vi "Test HighFrequency Client Connection.vi"() -> ()   [LabVIEW 2013]
uses:
  <vilib>/LabVIEW Open Source Project/MQTT Control Packets/Control Packets/CONNACK/Connect Return Code -- enum.ctl
  source/Server class/Server.lvclass/Server.ctl
  <vilib>/LabVIEW Open Source Project/MQTT Client/Client class/Client.lvclass/Client.ctl
  <vilib>/LabVIEW Open Source Project/MQTT Control Packets/Control Packets/PUBLISH/PUBLISH.lvclass
  source/Server class/Server.lvclass
  <vilib>/LabVIEW Open Source Project/MQTT Connection/MQTT_Base/Base Class/MQTT_Base.lvclass
  <vilib>/LabVIEW Open Source Project/MQTT Client/Client class/Client.lvclass
  <vilib>/LabVIEW Open Source Project/MQTT TCP Connection/MQTT_TCP/Connection/TCPConnection.lvclass
  <vilib>/LabVIEW Open Source Project/MQTT Control Packets/Control Packets/CONNACK/CONNACK.lvclass
panel:
  out "Start timed out":bool
  out "NO RESPONSE":bool
  out "Stop timed out?":bool
  out "Stop":dbl format="%.06f"
  out "Connect":dbl format="%.06f"
  out "Start":dbl format="%.06f"
  out "STOPPING":bool
  out "Waveform Chart":T1(graph)
  out "Loop period (s)":dbl format="%.06f"
  out "client Outgoing ID Request":i32
  out "Process Response":i32
  out "Process Incoming ID Request":i32
  out "Process Status":T2=enum."Server Unavailable"
  out "error server":errorcluster
  out "Client Status":T2=enum."Server Unavailable"
  out "error client process":errorcluster
  out "NbConnections":u32
  out "error client consumer":errorcluster
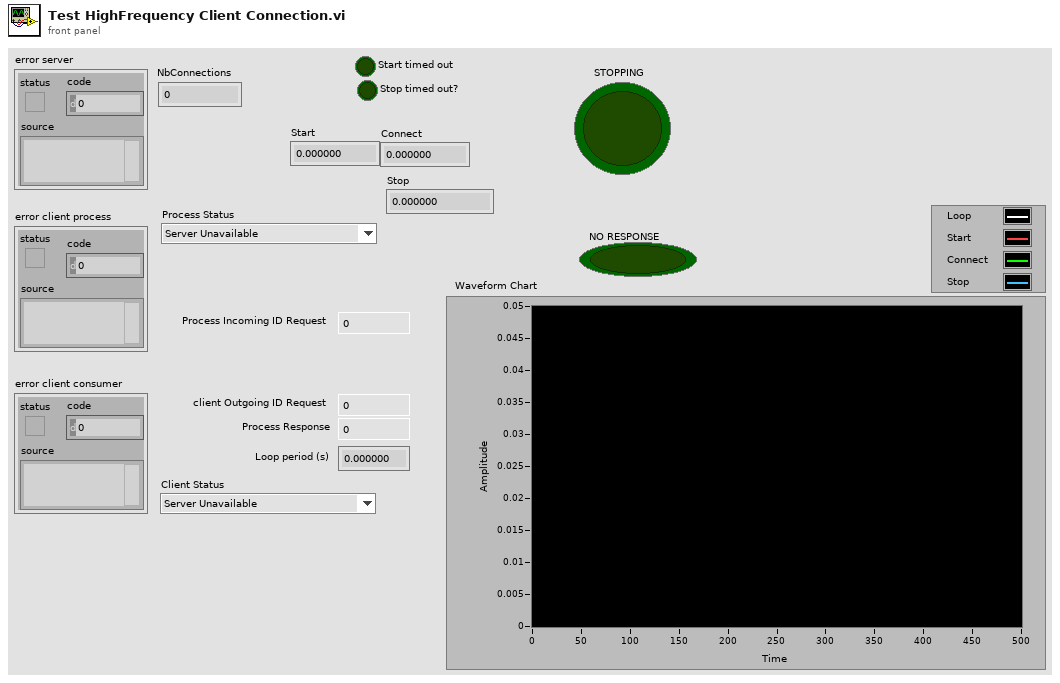
[diagram p1: front panel]
types:
  T1 = cluster{dbl, "elapsed (s)":dbl, "elapsed (s)":dbl, "elapsed (s)":dbl}
  T2 = typedef "MQTT_Control_Packets.lvlib/CONNACK.lvclass/Connect Return Code -- enum.ctl" = enum16{"Connection accepted", "Unacceptable protocol version", "Identifier Rejected", "Server Unavailable", "Bad Username or Password", "Not Authorized"}
  T3 = cluster{dbl, "elapsed (s)":dbl, "elapsed (s)":dbl, "elapsed (s)":dbl}[]
  T4 = typedef "MQTT Server.lvlib/Server.lvclass/Public Events -- cluster.ctl" = cluster{"NbConnections":refnum<user-event>}
  T5 = typedef "MQTT Client.lvlib/Client.lvclass/Public Events -- cluster.ctl" = cluster{"Connection Status":refnum<user-event>, "Connected":refnum<user-event>, "Application Message":refnum<user-event>}
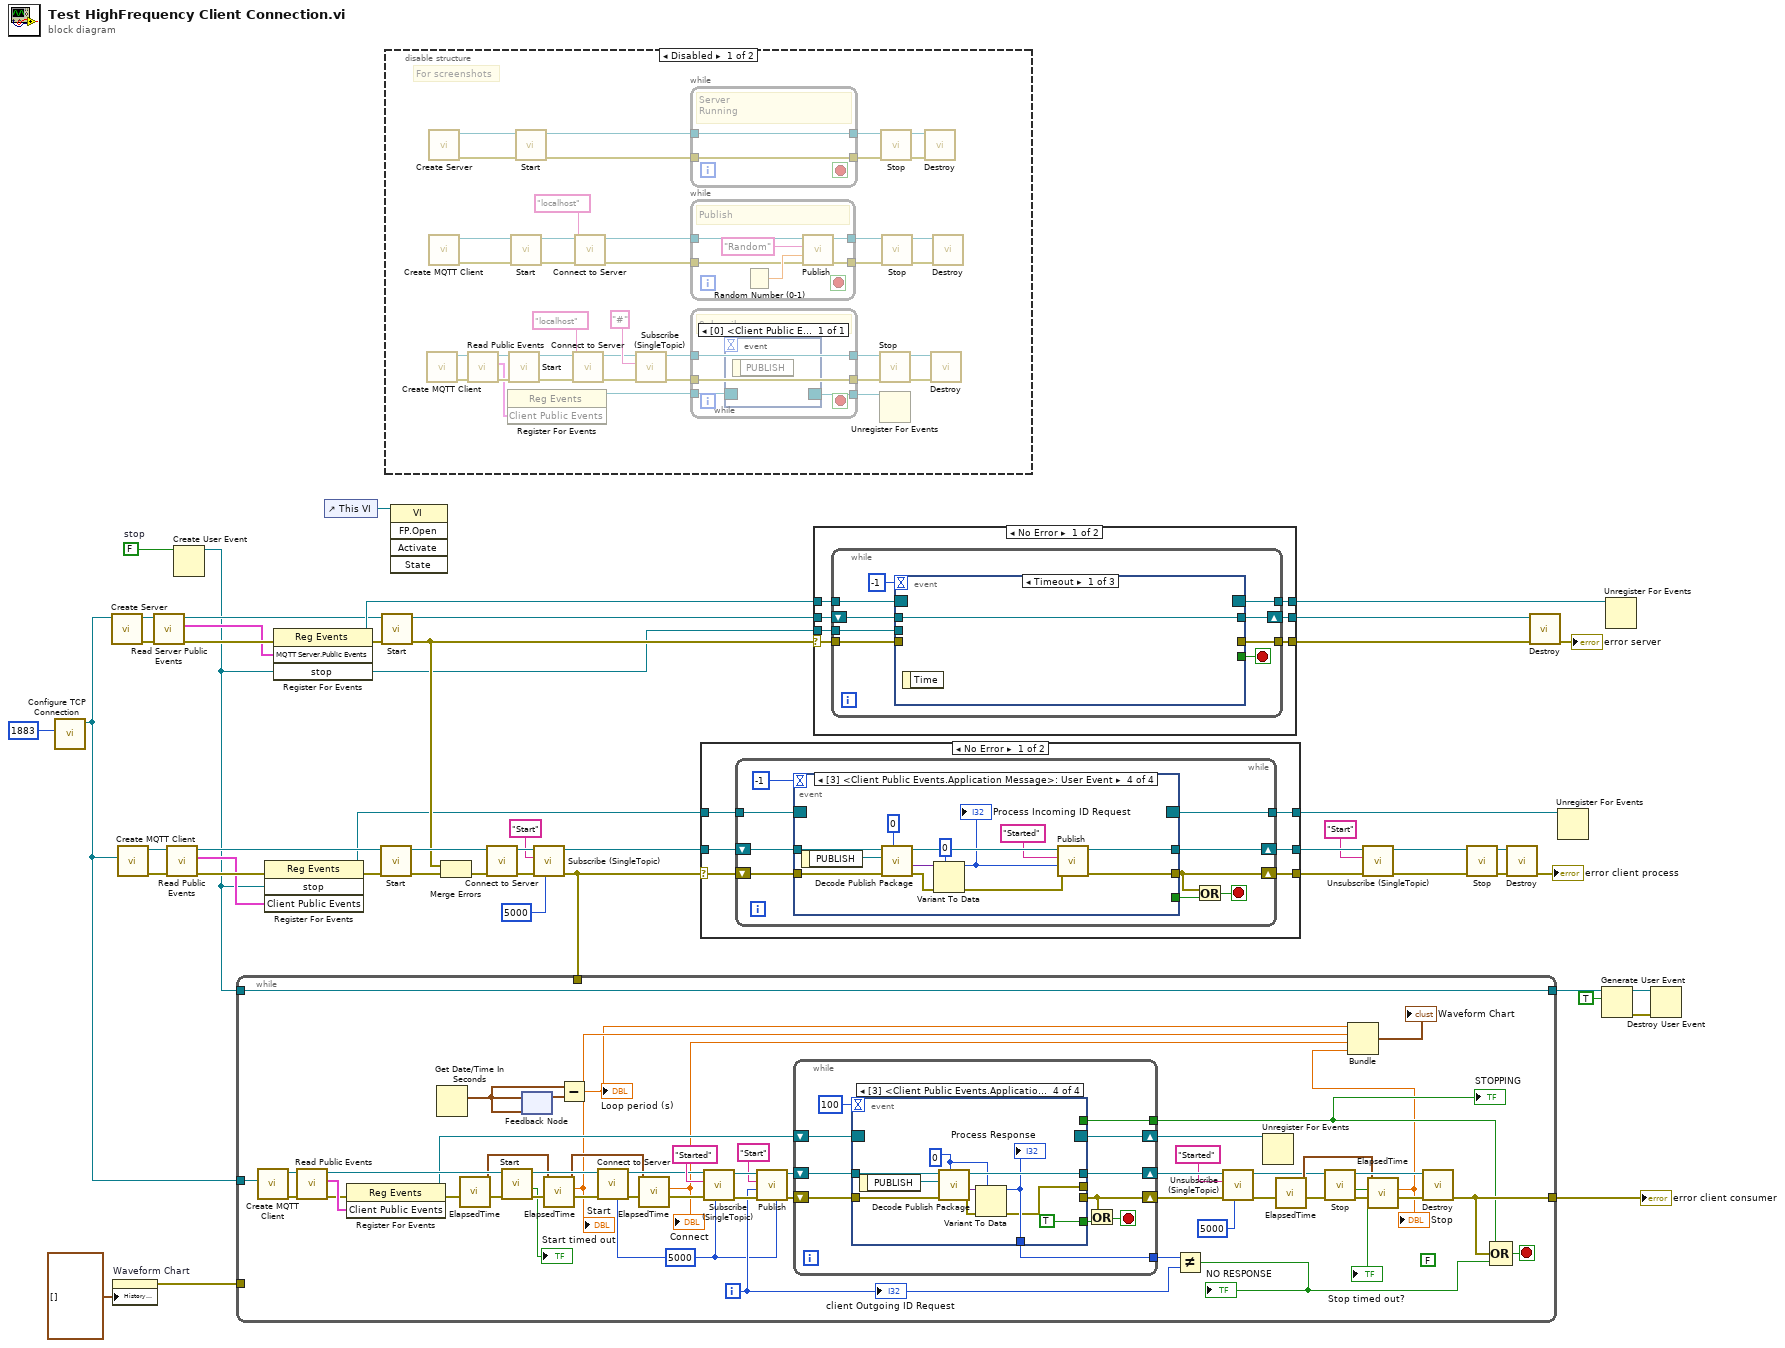
[diagram p0: block diagram]
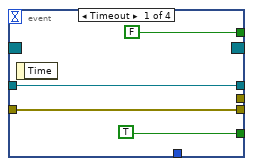
[diagram p2: hidden frame]
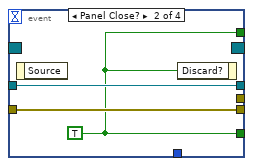
[diagram p3: hidden frame]
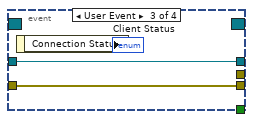
[diagram p4: hidden frame]
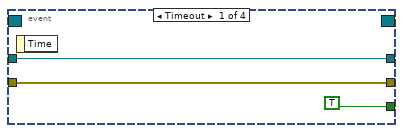
[diagram p5: hidden frame]
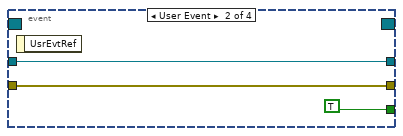
[diagram p6: hidden frame]
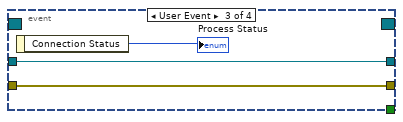
[diagram p7: hidden frame]
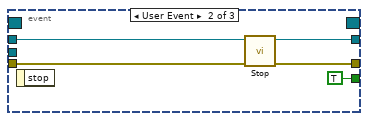
[diagram p10: hidden frame]
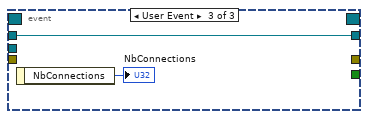
[diagram p11: hidden frame]
diagram:
  w33 = FALSE  # stop
  n1 = call <vilib>:"Configure TCP Connection.vi"("remote port (80)"=u16 1883) -> ("TCPConnection"=w2:refnum<class "TCPConnection.lvclass">)  [unwired: 9 in, 1 out]
  n2 = call "Create Server.vi"("Connection Configuration"=w2) -> ("error out"=w48:errorcluster, "Server"=w49:refnum<class "Server.lvclass">)  [unwired: 9 in]
  n3 = property on="Waveform Chart" class="WFChart (strict)"("History Data"=T3 []) -> (error out=w4:errorcluster)  [unwired: 2 in, 1 out]
  n4 = call <vilib>:"Create MQTT Client.vi"("Connection Configuration"=w2) -> ("error out"=w38:errorcluster, "Client out"=w37:refnum<class "Client.lvclass">)  [unwired: 9 in]
  n5 = call "Read Server Public Events.vi"("error in (no error)"=w48, "Server in"=w49) -> ("error out"=w47:errorcluster, "MQTT Server.Public Events"=w46:T4, "Server out"=w43:refnum<class "Server.lvclass">)  [unwired: 7 in]
  n6 = call <vilib>:"Read Public Events.vi"("error in (no error)"=w38, "Client in"=w37) -> ("error out"=w32:errorcluster, "Client Public Events"=w30:T5, "Client out"=w36:refnum<class "Client.lvclass">)  [unwired: 7 in]
  n7 = Create User Event(user event datatype=w33) -> (user event=w10:refnum<user-event>)  [unwired: 1 in, 1 out]
  n8 = register-events(error in=w32, w10, w30) -> (reference out=w22:refnum<event-registration>, error out=w31:errorcluster)  [unwired: 1 in]
  n9 = register-events(error in=w47, w46, w10) -> (reference out=w45:refnum<event-registration>, error out=w41:errorcluster)  [unwired: 1 in]
  n10 = control-ref of="This VI"() -> (w29:refnum<vi>)
  n11 = call <vilib>:"Start.vi"("error in (no error)"=w31, "MQTT_Base in"=w36) -> ("error out"=w34:errorcluster, "MQTT_Base out"=w35:refnum<class "Client.lvclass">)  [unwired: 7 in, 1 out]
  n12 = call <vilib>:"Start.vi"("error in (no error)"=w41, "MQTT_Base in"=w43) -> ("error out"=w27:errorcluster, "MQTT_Base out"=w42:refnum<class "Server.lvclass">)  [unwired: 7 in, 1 out]
  n13 = disable-structure shown="Disabled" {
    frame Disabled {
      # "For screenshots"
      n14 = call <vilib>:"Create MQTT Client.vi"() -> ("error out"=w55:errorcluster, "Client out"=w57:refnum<class "Client.lvclass">)  [unwired: 10 in]
      n15 = call "Create Server.vi"() -> ("error out"=w82:errorcluster, "Server"=w81:refnum<class "Server.lvclass">)  [unwired: 10 in]
      n16 = call <vilib>:"Create MQTT Client.vi"() -> ("error out"=w79:errorcluster, "Client out"=w80:refnum<class "Client.lvclass">)  [unwired: 10 in]
      n17 = call <vilib>:"Read Public Events.vi"("error in (no error)"=w55, "Client in"=w57) -> ("error out"=w54:errorcluster, "Client Public Events"=w53:T5, "Client out"=w56:refnum<class "Client.lvclass">)  [unwired: 7 in]
      n18 = register-events(w53) -> (reference out=w52:refnum<event-registration>)  [unwired: 2 in, 1 out]
      n19 = call <vilib>:"Start.vi"("error in (no error)"=w54, "MQTT_Base in"=w56) -> ("error out"=w72:errorcluster, "MQTT_Base out"=w73:refnum<class "Client.lvclass">)  [unwired: 7 in, 1 out]
      n20 = call <vilib>:"Start.vi"("error in (no error)"=w79, "MQTT_Base in"=w80) -> ("error out"=w86:errorcluster, "MQTT_Base out"=w85:refnum<class "Client.lvclass">)  [unwired: 7 in, 1 out]
      n21 = call <vilib>:"Start.vi"("error in (no error)"=w82, "MQTT_Base in"=w81) -> ("error out"=w64:errorcluster, "MQTT_Base out"=w66:refnum<class "Server.lvclass">)  [unwired: 7 in, 1 out]
      n22 = call <vilib>:"Connect to Server.vi"("error in (no error)"=w72, 10:"localhost" ("Topic Filter"), "Client in"=w73) -> ("error out"=w60:errorcluster, "Client out"=w61:refnum<class "Client.lvclass">)  [unwired: 5 in, 2 out]
      n23 = call <vilib>:"Connect to Server.vi"("error in (no error)"=w86, 10:"localhost" ("Topic Filter"), "Client in"=w85) -> ("error out"=w68:errorcluster, "Client out"=w71:refnum<class "Client.lvclass">)  [unwired: 5 in, 2 out]
      n24 = call <vilib>:"Subscribe (SingleTopic).vi"("error in (no error)"=w60, "Topic Filter"="#", "MQTT_Base in"=w61) -> ("error out"=w58:errorcluster, "MQTT_Base out"=w59:refnum<class "Client.lvclass">)  [unwired: 6 in, 1 out]
      n25 = while {
        tunnel: [w100] -> w67
        tunnel: w66 -> [w100]
        tunnel: w64 -> [w99]
        tunnel: [w99] -> w65
        stop <- _ stop-if-true
        # "Server\nRunning"
      }
      n26 = while {
        tunnel: w71 -> [w96]
        tunnel: [w95] -> w70
        tunnel: [w94] -> w69
        tunnel: w68 -> [w93]
        stop <- _ stop-if-true
        # "Publish"
        n27 = Random Number (0-1)() -> (number: 0 to 1=w98:dbl)
        n28 = call <vilib>:"Publish.vi"("error in (no error)"=w93, "Payload"=w98, "Topic Name (empty: Payload name)"="Random", "Client in"=w96) -> ("error out"=w94:errorcluster, "Client out"=w95:refnum<class "Client.lvclass">)  [unwired: 5 in, 1 out]
      }
      n29 = while {
        tunnel: [w92] -> w62
        tunnel: w59 -> [w92]
        tunnel: w58 -> [w91]
        tunnel: [w91] -> w63
        tunnel: w52 -> [w90]
        tunnel: [w89] -> w51
        stop <- _ stop-if-true
        # "Subscribe"
        n30 = event shown="[0] <Client Public Events.Application Message>: User Event" {
          selector: w90 -> [_]
          dyn-events: [_] -> w89
          timeout: _ -> [_]
          event User Event {
            n31 = event-data() -> ()  [unwired: 1 in, 1 out]
          }
        }
      }
      n32 = call <vilib>:"Stop.vi"("error in (no error)"=w63, "MQTT_Base in"=w62) -> ("error out"=w75:errorcluster, "MQTT_Base out"=w76:refnum<class "Client.lvclass">)  [unwired: 7 in, 1 out]
      n33 = Unregister For Events(event registration refnum=w51) -> ()  [unwired: 1 in, 1 out]
      n34 = call <vilib>:"Stop.vi"("error in (no error)"=w65, "MQTT_Base in"=w67) -> ("error out"=w88:errorcluster, "MQTT_Base out"=w87:refnum<class "Server.lvclass">)  [unwired: 7 in, 1 out]
      n35 = call <vilib>:"Stop.vi"("error in (no error)"=w69, "MQTT_Base in"=w70) -> ("error out"=w84:errorcluster, "MQTT_Base out"=w83:refnum<class "Client.lvclass">)  [unwired: 7 in, 1 out]
      n36 = call <vilib>:"Destroy.vi"("error in (no error)"=w88, "MQTT_Base in"=w87) -> ()  [unwired: 8 in, 2 out]
      n37 = call <vilib>:"Destroy.vi"("error in (no error)"=w75, "MQTT_Base in"=w76) -> ()  [unwired: 8 in, 2 out]
      n38 = call <vilib>:"Destroy.vi"("error in (no error)"=w84, "MQTT_Base in"=w83) -> ()  [unwired: 8 in, 2 out]
    }
    frame Enabled {
    }
  }
  n39 = invoke class="VI" method="FP.Open"(reference=w29) -> ()  [unwired: 4 in, 5 out]
  n40 = Merge Errors(w27, w34) -> (w39:errorcluster)
  n41 = call <vilib>:"Connect to Server.vi"("error in (no error)"=w39, "Client in"=w35) -> ("error out"=w25:errorcluster, "Client out"=w26:refnum<class "Client.lvclass">)  [unwired: 6 in, 2 out]
  n42 = call <vilib>:"Subscribe (SingleTopic).vi"("timeout (100ms)"=5000, "error in (no error)"=w25, "Topic Filter"="Start", "MQTT_Base in"=w26) -> ("error out"=w11:errorcluster, "MQTT_Base out"=w23:refnum<class "Client.lvclass">)  [unwired: 5 in, 1 out]
  n43 = while {
    tunnel: [w134] -> w12
    tunnel: w11 -> [_]
    tunnel: [w132] -> w9
    tunnel: w10 -> [w132]
    tunnel: w4 -> [_]
    tunnel: w2 -> [w104]
    i -> [w133]
    stop <- w135 stop-if-true
    w103 = 5000 ("timeout (100ms)")
    (unwired) FALSE
    n44 = call <vilib>:"Create MQTT Client.vi"("Connection Configuration"=w104) -> ("error out"=w151:errorcluster, "Client out"=w152:refnum<class "Client.lvclass">)  [unwired: 9 in]
    n45 = call <vilib>:"Read Public Events.vi"("error in (no error)"=w151, "Client in"=w152) -> ("error out"=w146:errorcluster, "Client Public Events"=w147:T5, "Client out"=w150:refnum<class "Client.lvclass">)  [unwired: 7 in]
    n46 = register-events(error in=w146, w147) -> (reference out=w145:refnum<event-registration>, error out=w128:errorcluster)  [unwired: 1 in]
    n47 = Get Date/Time In Seconds() -> (seconds since 1Jan1904=w130:timestamp)
    n48 = call <vilib>:"ElapsedTime.vi"("error in"=w128) -> ("error out"=w127:errorcluster, "current time"=w124:timestamp)  [unwired: 8 in, 1 out]
    n49 = call <vilib>:"Start.vi"("error in (no error)"=w127, "MQTT_Base in"=w150) -> ("error out"=w125:errorcluster, "timed out?"=→"Start timed out":bool, "MQTT_Base out"=w149:refnum<class "Client.lvclass">)  [unwired: 7 in]
    n50 = feedback-in #1(w130) -> ()
    n51 = feedback #1(w130) -> (w131:timestamp)
    n52 = call <vilib>:"ElapsedTime.vi"("error in"=w125, "compare time"=w124) -> ("error out"=w126:errorcluster, "elapsed (s)"=w116:dbl, "current time"=w121:timestamp)  [unwired: 7 in]
    "Start" <- w116
    n53 = Subtract(x=w130, y=w131) -> (x-y=w113:dbl)
    "Loop period (s)" <- w113
    n54 = call <vilib>:"Connect to Server.vi"("timeout (2000 ms)"=w103, "error in (no error)"=w126, "Client in"=w149) -> ("error out"=w123:errorcluster, "Client out"=w142:refnum<class "Client.lvclass">)  [unwired: 5 in, 2 out]
    n55 = call <vilib>:"ElapsedTime.vi"("error in"=w123, "compare time"=w121) -> ("error out"=w122:errorcluster, "elapsed (s)"=w115:dbl)  [unwired: 7 in, 1 out]
    "Connect" <- w115
    n56 = call <vilib>:"Subscribe (SingleTopic).vi"("timeout (100ms)"=w103, "error in (no error)"=w122, "Topic Filter"="Started", "MQTT_Base in"=w142) -> ("error out"=w141:errorcluster, "MQTT_Base out"=w140:refnum<class "Client.lvclass">)  [unwired: 5 in, 1 out]
    n57 = call <vilib>:"Publish.vi"("timeout (1000ms)"=w103, "error in (no error)"=w141, "Payload"=w133, "Topic Name (empty: Payload name)"="Start" ("Topic Filter"), "Client in"=w140) -> ("error out"=w138:errorcluster, "Client out"=w139:refnum<class "Client.lvclass">)  [unwired: 4 in, 1 out]
    n58 = while {
      shift-right: [w161] -> w109
      shift-left: w139 -> [w157]
      shift-right: [w162] -> w144
      shift-left: w145 -> [w163]
      shift-right: [w160] -> w107
      shift-left: w138 -> [w156]
      tunnel: [w154] -> w136
      tunnel: [w153] -> w129
      stop <- w155 stop-if-true
      n59 = event shown="[3] <Client Public Events.Application Message>: User Event" {
        selector: w163 -> [_ _ _ _]
        dyn-events: [_ _ _ _] -> w162
        timeout: 100 -> [_ _ _ _]
        tunnel: w157 -> [w166 w170 w172 w182]
        tunnel: [w166 w170 w172 w180] -> w161
        tunnel: [w165 w169 w171 _] -> w160
        tunnel: w156 -> [w165 w169 w171 w179]
        tunnel: [TRUE w168 _ TRUE] -> w159
        tunnel: [_ _ _ w175] -> w154
        tunnel: [FALSE w168 _ _] -> w153
        tunnel: [_ _ _ w174] -> _
        event Timeout {
          n60 = event-data() -> ()  [unwired: 1 in, 1 out]
        }
        event Panel Close? {
          w168 = TRUE
          n61 = event-data() -> ()  [unwired: 1 in, 1 out]
          n62 = event-data("Discard?"=w168) -> ()  [unwired: 1 in, 1 out]
        }
        event User Event {
          n63 = event-data() -> ("Connection Status"=→"Client Status":T2)  [unwired: 1 in]
        }
        event User Event {
          w178 = 0
          n64 = event-data() -> ("PUBLISH"=w183:refnum<class "PUBLISH.lvclass">)  [unwired: 1 in]
          n65 = call <vilib>:"Decode Publish Package.vi"("Type"=w178, "error in (no error)"=w179, "PUBLISH"=w183, "MQTT_Base in"=w182) -> ("error out"=w177:errorcluster, "Payload"=w181:variant, "MQTT_Base out"=w180:refnum<class "Client.lvclass">)  [unwired: 4 in, 1 out]
          n66 = Variant To Data(error in=w177, type=w178, Variant=w181) -> (data=w175:i32, error out=w174:errorcluster)
          "Process Response" <- w175
        }
      }
      n67 = Or(x=w160, y=w159) -> (x .or. y?=w155:bool)
    }
    "STOPPING" <- w129
    n68 = Not Equal?(x=w136, y=w133) -> (x != y?=w110:bool)
    "NO RESPONSE" <- w110
    n69 = call <vilib>:"Unsubscribe (SingleTopic).vi"("timeout (100ms)"=5000, "error in (no error)"=w107, "Topic Filter"="Started", "MQTT_Base in"=w109) -> ("error out"=w106:errorcluster, "MQTT_Base out"=w108:refnum<class "Client.lvclass">)  [unwired: 5 in, 1 out]
    n70 = Unregister For Events(event registration refnum=w144) -> ()  [unwired: 1 in, 1 out]
    n71 = call <vilib>:"ElapsedTime.vi"("error in"=w106) -> ("error out"=w120:errorcluster, "current time"=w117:timestamp)  [unwired: 8 in, 1 out]
    n72 = call <vilib>:"Stop.vi"("error in (no error)"=w120, "MQTT_Base in"=w108) -> ("error out"=w118:errorcluster, "timed out?"=→"Stop timed out?":bool, "MQTT_Base out"=w148:refnum<class "Client.lvclass">)  [unwired: 7 in]
    n73 = call <vilib>:"ElapsedTime.vi"("error in"=w118, "compare time"=w117) -> ("error out"=w119:errorcluster, "elapsed (s)"=w114:dbl)  [unwired: 7 in, 1 out]
    "Stop" <- w114
    n74 = Bundle(w113, "elapsed (s)"=w116, "elapsed (s)"=w115, "elapsed (s)"=w114) -> (→"Waveform Chart":T1)  [unwired: 1 in]
    n75 = call <vilib>:"Destroy.vi"("error in (no error)"=w119, "MQTT_Base in"=w148) -> ("error out"=w134:errorcluster)  [unwired: 8 in, 1 out]
    n76 = Compound Arithmetic op=OR(w129, w134, w110) -> (w135:bool)
    "client Outgoing ID Request" <- w133
  }
  "error client consumer" <- w12
  n77 = case shown="No Error" w11 {
    selector: w11 -> [w184 w221]
    tunnel: w22 -> [w189 w223]
    tunnel: [w188 w223] -> w18
    tunnel: w23 -> [w187 w222]
    tunnel: [w186 w222] -> w16
    tunnel: [w185 w221] -> w14
    frame No Error {
      n78 = while {
        tunnel: w189 -> [w198]
        tunnel: [w197] -> w188
        shift-right: [w195] -> w186
        shift-left: w187 -> [w196]
        shift-right: [w192] -> w185
        shift-left: w184 -> [w194]
        stop <- w193 stop-if-true
        n79 = event shown="[3] <Client Public Events.Application Message>: User Event" {
          selector: w198 -> [_ _ _ _]
          dyn-events: [_ _ _ _] -> w197
          timeout: -1 -> [_ _ _ _]
          tunnel: w196 -> [w200 w203 w206 w219]
          tunnel: [w200 w203 w206 w212] -> w195
          tunnel: [w199 w202 w205 w208] -> w192
          tunnel: w194 -> [w199 w202 w205 w216]
          tunnel: [TRUE TRUE _ _] -> w191
          event Timeout {
            n80 = event-data() -> ()  [unwired: 1 in, 1 out]
          }
          event User Event {
            n81 = event-data() -> ()  [unwired: 1 in, 1 out]
          }
          event User Event {
            n82 = event-data() -> ("Connection Status"=→"Process Status":T2)  [unwired: 1 in]
          }
          event User Event {
            n83 = event-data() -> ("PUBLISH"=w220:refnum<class "PUBLISH.lvclass">)  [unwired: 1 in]
            n84 = call <vilib>:"Decode Publish Package.vi"("Type"=0, "error in (no error)"=w216, "PUBLISH"=w220, "MQTT_Base in"=w219) -> ("error out"=w215:errorcluster, "Payload"=w218:variant, "MQTT_Base out"=w213:refnum<class "Client.lvclass">)  [unwired: 4 in, 1 out]
            n85 = Variant To Data(error in=w215, type=0, Variant=w218) -> (data=w210:i32, error out=w209:errorcluster)
            "Process Incoming ID Request" <- w210
            n86 = call <vilib>:"Publish.vi"("error in (no error)"=w209, "Payload"=w210, "Topic Name (empty: Payload name)"="Started" ("Topic Filter"), "Client in"=w213) -> ("error out"=w208:errorcluster, "Client out"=w212:refnum<class "Client.lvclass">)  [unwired: 5 in, 1 out]
          }
        }
        n87 = Or(x=w192, y=w191) -> (x .or. y?=w193:bool)
      }
    }
    frame Error {
    }
  }
  n88 = case shown="No Error" w27 {
    selector: w27 -> [w224 w248]
    tunnel: w42 -> [w230 w250]
    tunnel: [w229 w250] -> w50
    tunnel: w45 -> [w228 w249]
    tunnel: [w227 w249] -> w44
    tunnel: [w226 w248] -> w40
    tunnel: w10 -> [w225 _]
    frame No Error {
      n89 = while {
        shift-right: [w236] -> w229
        shift-left: w230 -> [w238]
        tunnel: w228 -> [w235]
        tunnel: [w234] -> w227
        tunnel: [w233] -> w226
        tunnel: w225 -> [w232]
        tunnel: w224 -> [w231]
        stop <- w237 stop-if-true
        n90 = event shown="[0] Timeout" {
          selector: w235 -> [_ _ _]
          dyn-events: [_ _ _] -> w234
          timeout: -1 -> [_ _ _]
          tunnel: w238 -> [w240 w245 w247]
          tunnel: [_ TRUE ("Discard?") _] -> w237
          tunnel: [w240 w244 w247] -> w236
          tunnel: [_ w243 _] -> w233
          tunnel: w232 -> [_ _ _]
          tunnel: w231 -> [_ w241 _]
          event Timeout {
            n91 = event-data() -> ()  [unwired: 1 in, 1 out]
          }
          event User Event {
            n92 = event-data() -> ()  [unwired: 1 in, 1 out]
            n93 = call <vilib>:"Stop.vi"("error in (no error)"=w241, "MQTT_Base in"=w245) -> ("error out"=w243:errorcluster, "MQTT_Base out"=w244:refnum<class "Server.lvclass">)  [unwired: 7 in, 1 out]
          }
          event User Event {
            n94 = event-data() -> ("NbConnections"=→"NbConnections":u32)  [unwired: 1 in]
          }
        }
      }
    }
    frame Error {
    }
  }
  n95 = call <vilib>:"Unsubscribe (SingleTopic).vi"("error in (no error)"=w14, "Topic Filter"="Start", "MQTT_Base in"=w16) -> ("error out"=w15:errorcluster, "MQTT_Base out"=w17:refnum<class "Client.lvclass">)  [unwired: 6 in, 1 out]
  n96 = call <vilib>:"Stop.vi"("error in (no error)"=w15, "MQTT_Base in"=w17) -> ("error out"=w20:errorcluster, "MQTT_Base out"=w21:refnum<class "Client.lvclass">)  [unwired: 7 in, 1 out]
  n97 = call <vilib>:"Destroy.vi"("error in (no error)"=w20, "MQTT_Base in"=w21) -> ("error out"=→"error client process":errorcluster)  [unwired: 8 in, 1 out]
  n98 = call <vilib>:"Destroy.vi"("error in (no error)"=w40, "MQTT_Base in"=w50) -> ("error out"=→"error server":errorcluster)  [unwired: 8 in, 1 out]
  n99 = Unregister For Events(event registration refnum=w18) -> ()  [unwired: 1 in, 1 out]
  n100 = Generate User Event(user event=w9, event data cluster=TRUE ("event data")) -> (user event out=w7:refnum<user-event>, error out=w8:errorcluster)  [unwired: 2 in]
  n101 = Unregister For Events(event registration refnum=w44) -> ()  [unwired: 1 in, 1 out]
  n102 = Destroy User Event(user event=w7, error in=w8) -> ()  [unwired: 1 out]
